vi "DegToRad.vi"(11 "Degrees":dbl) -> (3 "Radians":dbl)   [LabVIEW 2016]
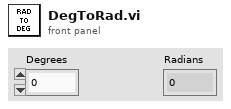
[diagram p1: front panel]
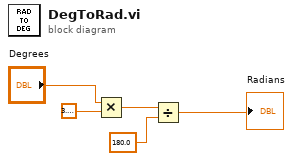
[diagram p0: block diagram]
diagram:
  n1 = Multiply(x="Degrees", y=3.141592653589793) -> (x*y=w4:dbl)
  n2 = Divide(x=w4, y=180.0) -> (x/y=→"Radians":dbl)
